vi "Combustion Stability Analysis.vi"() -> ()   [LabVIEW 2021]
uses:
  <vilib>/Utility/file.llb/Read Delimited Spreadsheet (string).vi
  <vilib>/Utility/file.llb/Read Delimited Spreadsheet (DBL).vi
panel:
  out "P-V Graph 3":cluster{" Total volume Vd":dbl[], dbl[]}(graph)
  out "Cycle Number":i32
  out "COV IMEP":dbl[](graph)
  out "COV Pmax":dbl[](graph)
  out "IMEP":dbl[](graph)
  out "P-V Graph 2":cluster{" Total volume Vd":dbl[], dbl[]}(graph)
  out "Data from file":dbl[][](array[numeric])
  out "CAmax per cycle":i32[](graph)
  out "CA(dp/dCA)max Graph":i32[](graph)
  out "(dp/dCA)max Graph  2":dbl[](graph)
  out "Pmax per cycle":dbl[](graph)
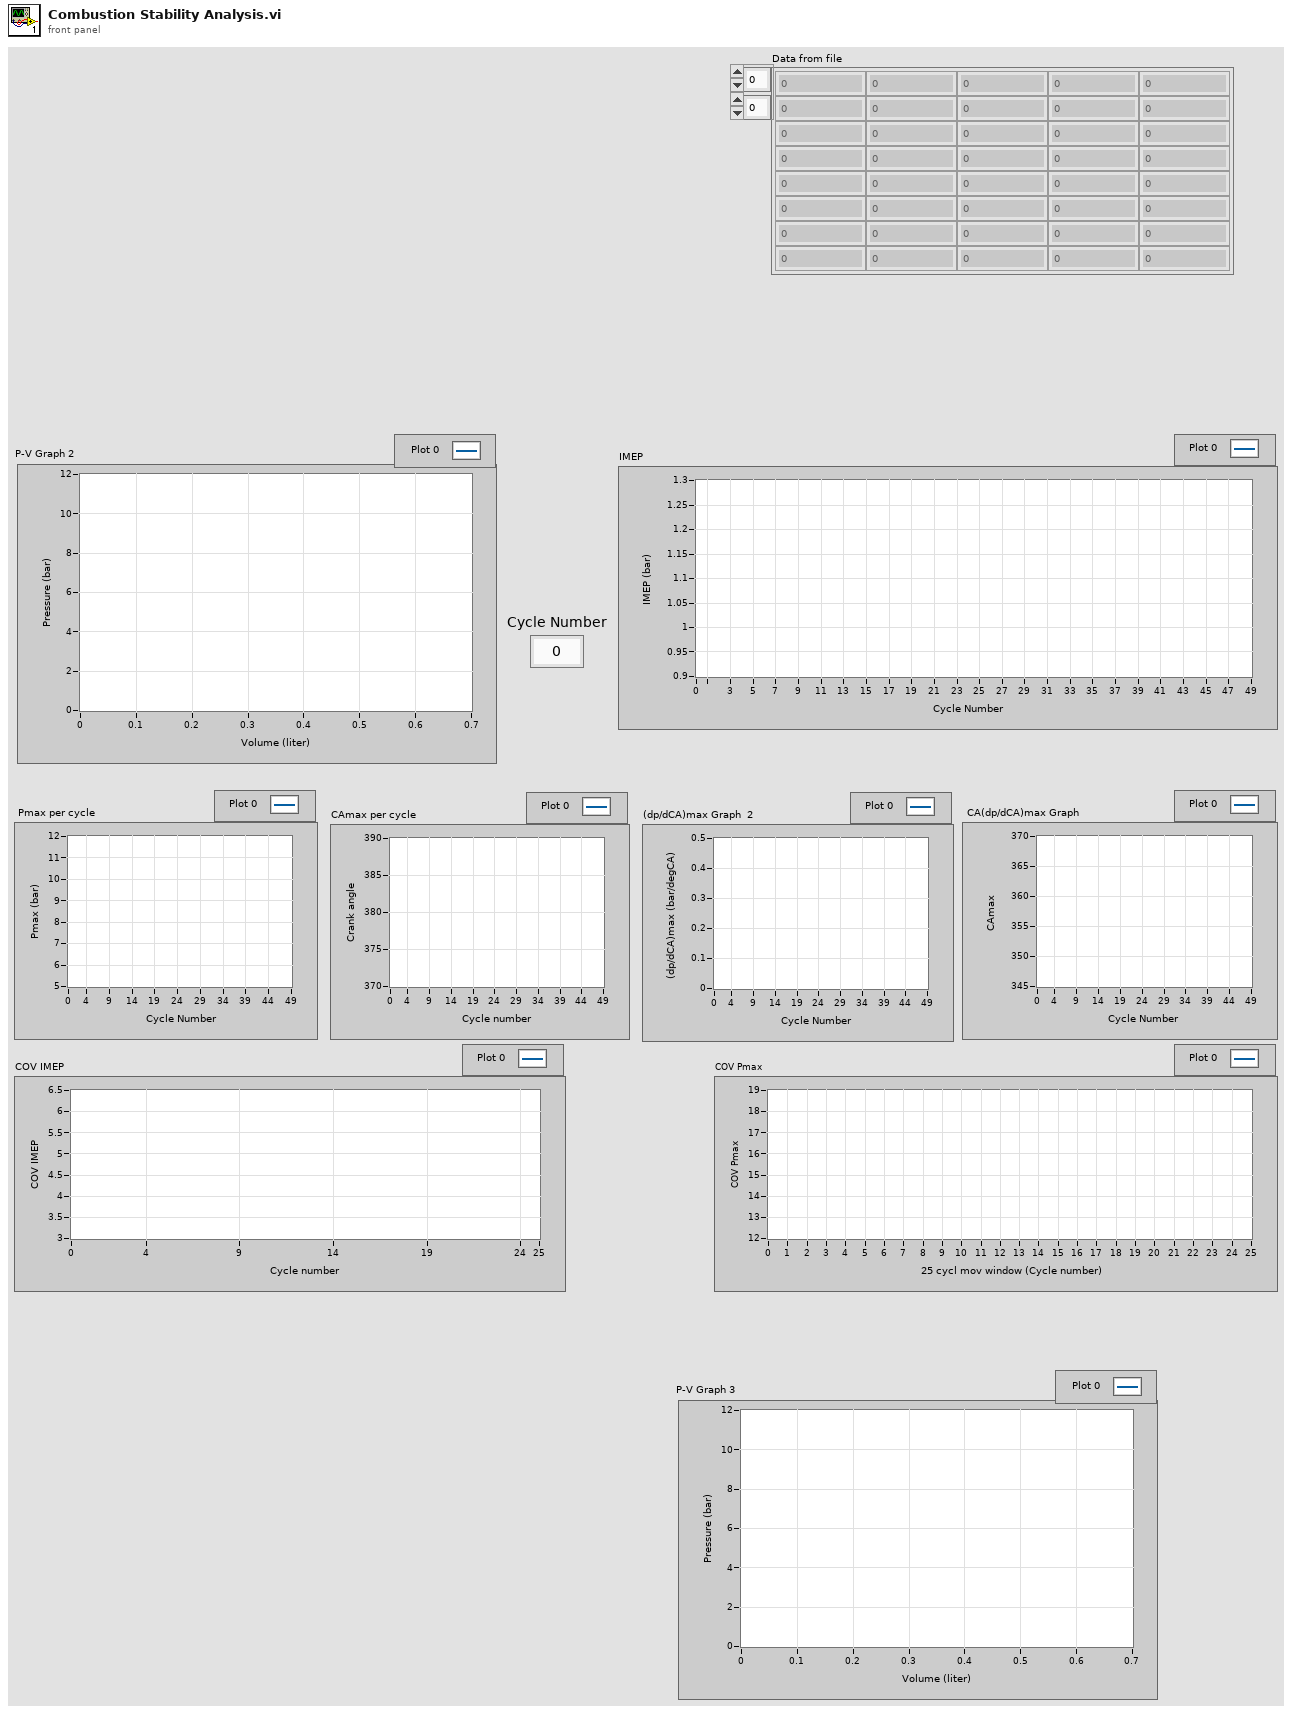
[diagram p1: front panel]
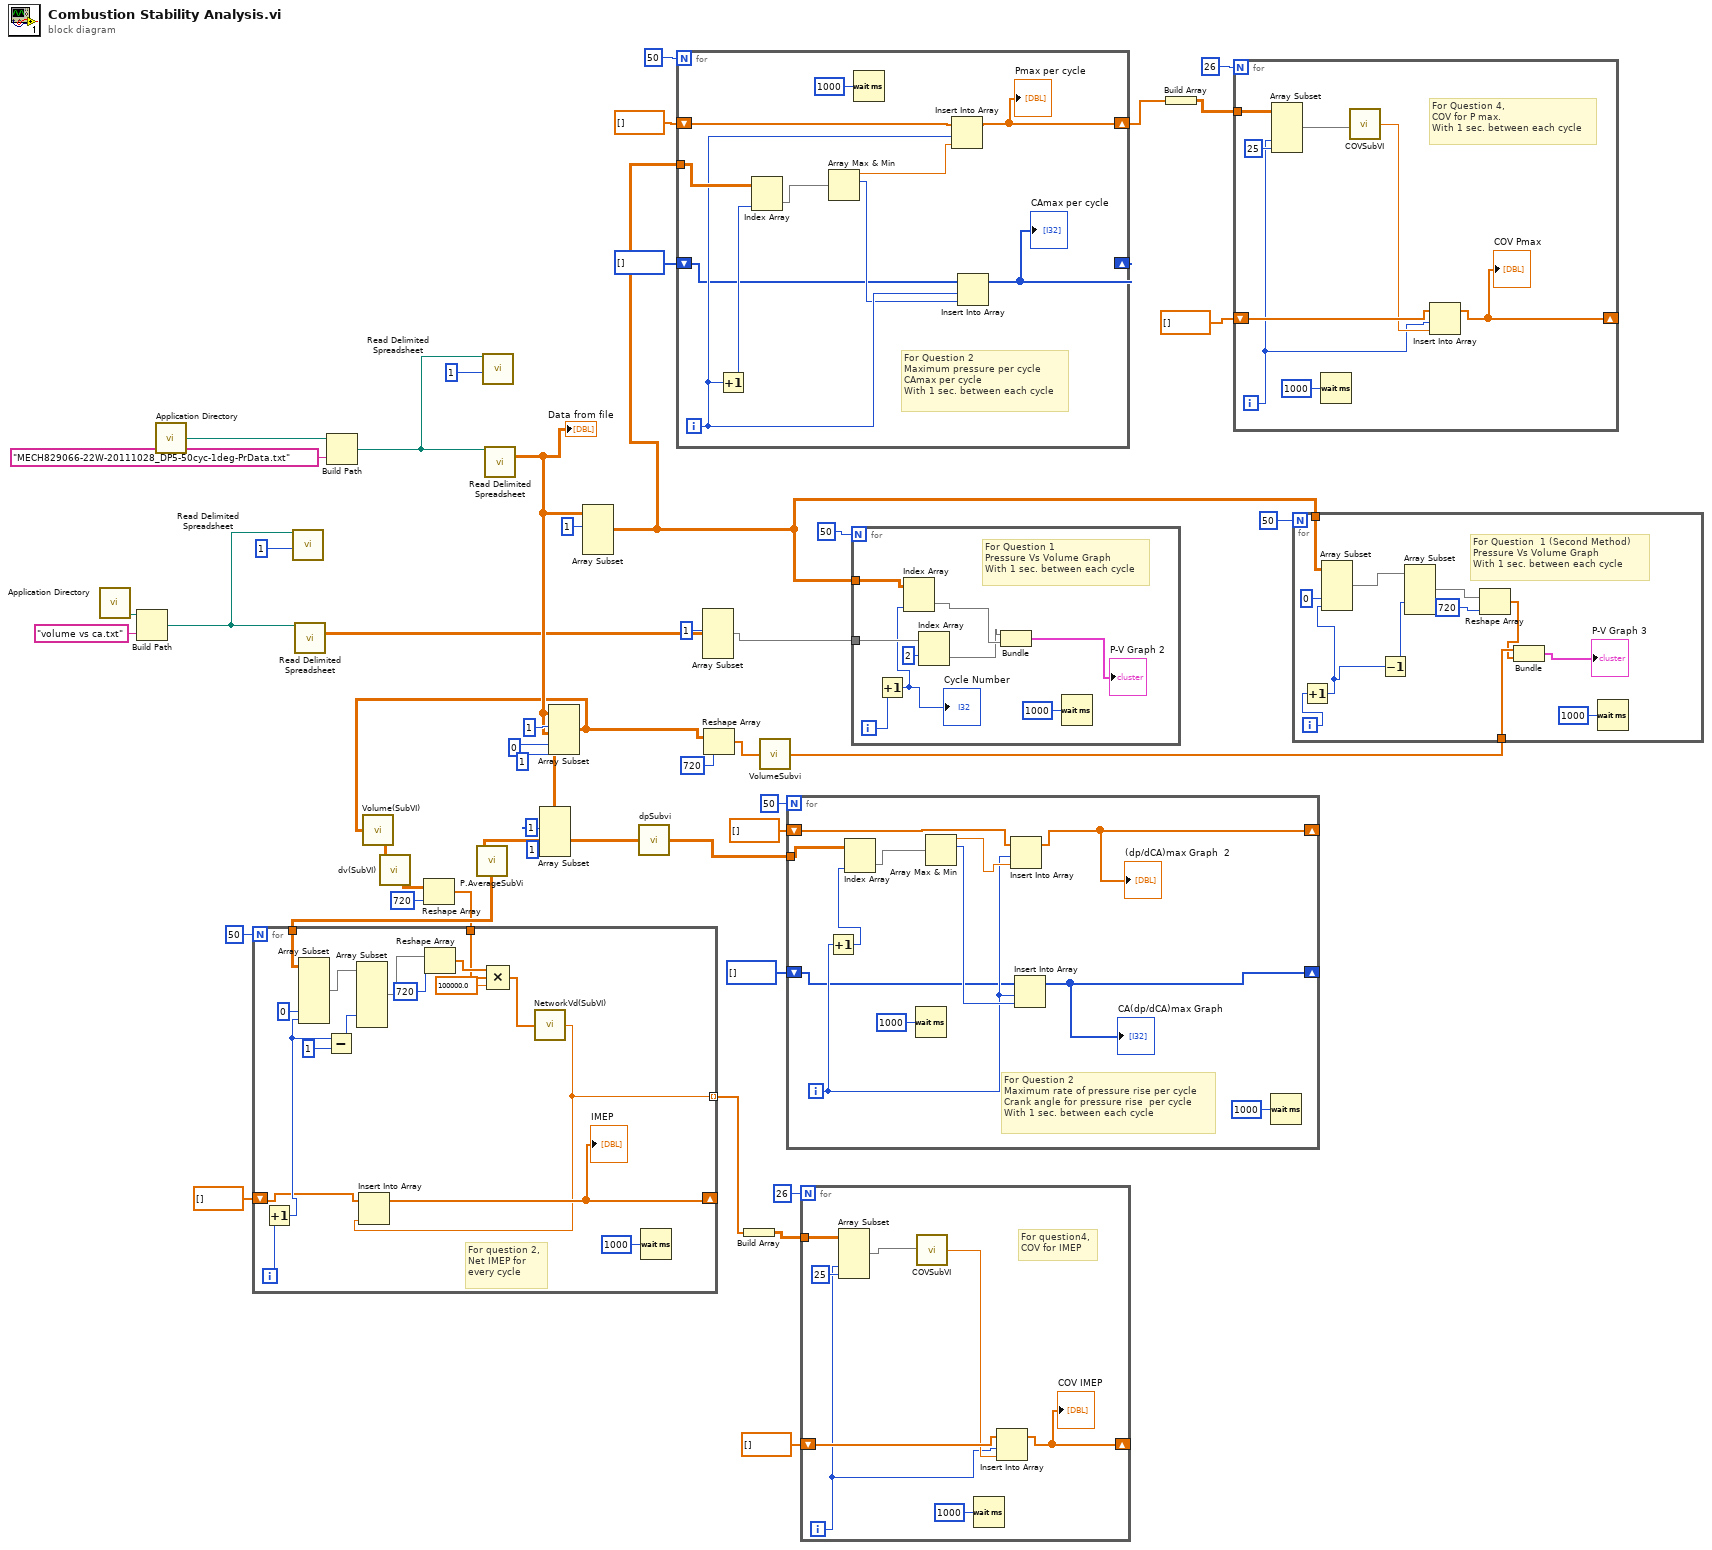
[diagram p0: block diagram]
diagram:
  n1 = call <vilib>:"Application Directory.vi"() -> ("Application Directory"=w25:path)
  n2 = Build Path(base path=w25, name or relative path="volume vs ca.txt") -> (appended path=w27:path)
  n3 = call <vilib>:"Application Directory.vi"() -> ("Application Directory"=w48:path)
  n4 = call-poly <vilib>:"Read Delimited Spreadsheet.vi"("file path (dialog if empty)"=w27, "number of rows (all:-1)"=1) -> ()  [unwired: 8 in, 6 out]
  n5 = call-poly <vilib>:"Read Delimited Spreadsheet.vi"("file path (dialog if empty)"=w27) -> ("all rows"=w24:dbl[][])  [unwired: 9 in, 5 out]
  n6 = Build Path(base path=w48, name or relative path="MECH829066-22W-20111028_DP5-50cyc-1deg-PrData.txt") -> (appended path=w46:path)
  n7 = call-poly <vilib>:"Read Delimited Spreadsheet.vi"("file path (dialog if empty)"=w46, "number of rows (all:-1)"=1) -> ()  [unwired: 8 in, 6 out]
  n8 = call-poly <vilib>:"Read Delimited Spreadsheet.vi"("file path (dialog if empty)"=w46) -> ("all rows"=w33:dbl[][])  [unwired: 9 in, 5 out]
  "Data from file" <- w33
  n9 = Array Subset "Array Subset"(array=w33, index (row)=1 ("index"), index (col)=1 ("index")) -> (w19:dbl[][])  [unwired: 2 in]
  n10 = call "P.AverageSubVi.vi"("Array"=w19) -> ("output array"=w30:dbl[][][])
  n11 = Array Subset "Array Subset"(array=w33, index (row)=1 ("index"), index (col)=0 ("index"), length (col)=1 ("length")) -> (w5:dbl[][])  [unwired: 1 in]
  n12 = call "Volume(SubVI).vi"("Array in"=w5) -> ("Array out"=w11:dbl[][])
  n13 = call "dv(SubVI).vi"("Array in"=w11) -> ("Array"=w10:dbl[][][])
  n14 = Reshape Array(w10, 720 ("dimension size")) -> (w8:dbl[])
  n15 = for {
    N: 50 -> [_]
    tunnel: w30 -> [w65]
    shift-right: [w52] -> _
    shift-left: dbl[] [] -> [w53]
    tunnel: [w51] -> w14 mode=indexing
    tunnel: w8 -> [w50]
    i -> [w63]
    # "For question 2,\nNet IMEP for\nevery cycle"
    n16 = Increment(x=w63) -> (x+1=w61:i32)
    n17 = Array Subset "Array Subset"(array=w65, index (dim 2)=0 ("index"), length (dim 2)=w61) -> (w62:dbl[][][])  [unwired: 4 in]
    n18 = Subtract(x=w61, y=1) -> (x-y=w60:i32)
    n19 = Array Subset(array=w62, index (dim 2)=w60) -> (w58:dbl[][][])  [unwired: 5 in]
    n20 = Reshape Array "Reshape Array"(w58, 720 ("dimension size")) -> (w55:dbl[])
    n21 = Compound Arithmetic op=MULTIPLY(w55, w50, 100000.0 ("value")) -> (w54:dbl[])
    n22 = call "NetworkVd(SubVI).vi"("Array"=w54) -> ("Numeric"=w51:dbl)
    n23 = Insert Into Array "Insert Into Array"(array=w53, new element=w51) -> (w52:dbl[])  [unwired: 1 in]
    "IMEP" <- w52
    n24 = Wait (ms)(milliseconds to wait=u32 1000) -> ()  [unwired: 1 out]
  }
  n25 = Array Subset "Array Subset"(array=w33, index (row)=1 ("index")) -> (w6:dbl[][])  [unwired: 3 in]
  n26 = call "dpSubvi.vi"("Array"=w19) -> ("output array"=w29:dbl[][])
  n27 = for {
    N: 50 -> [_]
    tunnel: w6 -> [w76]
    shift-right: [w72] -> w17
    shift-left: dbl[] [] -> [w73]
    shift-right: [w67] -> _
    shift-left: i32[] [] -> [w68]
    i -> [w70]
    # "For Question 2\nMaximum pressure per cycle\nCAmax per cycle\nWith 1 sec. between each cycle"
    n28 = Increment(x=w70) -> (x+1=w75:i32)
    n29 = Index Array "Index Array"(array=w76, index (col)=w75) -> (element=w74:dbl[])  [unwired: 1 in]
    n30 = Array Max & Min(array=w74) -> (max value=w71:dbl, max index (indices)=w69:i32)  [unwired: 2 out]
    n31 = Wait (ms)(milliseconds to wait=u32 1000) -> ()  [unwired: 1 out]
    n32 = Insert Into Array "Insert Into Array"(array=w73, index=w70, new element=w71) -> (w72:dbl[])
    "Pmax per cycle" <- w72
    n33 = Insert Into Array "Insert Into Array"(array=w68, index=w70, new element=w69) -> (w67:i32[])
    "CAmax per cycle" <- w67
  }
  n34 = Array Subset "Array Subset"(array=w24, index (row)=1 ("index")) -> (w22:dbl[][])  [unwired: 3 in]
  n35 = Reshape Array(w5, 720 ("dimension size")) -> (w3:dbl[])
  n36 = Build Array(w14) -> (w13:dbl[][])
  n37 = call "VolumeSubvi.vi"("Array"=w3) -> ("Total volume Vd"=w2:dbl[])
  n38 = for {
    N: 50 -> [_]
    shift-right: [w85] -> _
    shift-left: dbl[] [] -> [w86]
    shift-right: [w81] -> _
    shift-left: i32[] [] -> [w82]
    tunnel: w29 -> [w80]
    i -> [w83]
    # "For Question 2\nMaximum rate of pressure rise per cycle\nCrank angle for pressure rise  per cycle\nWith 1 sec. between each cycle"
    n39 = Increment(x=w83) -> (x+1=w79:i32)
    n40 = Index Array "Index Array"(array=w80, index (col)=w79) -> (element=w78:dbl[])  [unwired: 1 in]
    n41 = Wait (ms)(milliseconds to wait=u32 1000) -> ()  [unwired: 1 out]
    n42 = Array Max & Min(array=w78) -> (max value=w87:dbl, max index (indices)=w84:i32)  [unwired: 2 out]
    n43 = Insert Into Array "Insert Into Array"(array=w86, index=w83, new element=w87) -> (w85:dbl[])
    "(dp/dCA)max Graph  2" <- w85
    n44 = Insert Into Array "Insert Into Array"(array=w82, index=w83, new element=w84) -> (w81:i32[])
    "CA(dp/dCA)max Graph" <- w81
    n45 = Wait (ms)(milliseconds to wait=u32 1000) -> ()  [unwired: 1 out]
  }
  n46 = for {
    N: 26 -> [_]
    shift-right: [w93] -> _
    shift-left: dbl[] [] -> [w95]
    tunnel: w13 -> [w90]
    i -> [w91]
    # "For question4,\nCOV for IMEP"
    n47 = Array Subset "Array Subset"(array=w90, index (col)=w91, length (col)=25 ("length")) -> (w89:dbl[][])  [unwired: 2 in]
    n48 = call "COVSubVI.vi"("Array"=w89) -> ("Numeric"=w94:dbl)
    n49 = Wait (ms)(milliseconds to wait=u32 1000) -> ()  [unwired: 1 out]
    n50 = Insert Into Array(array=w95, index=w91, new element=w94) -> (w93:dbl[])
    "COV IMEP" <- w93
  }
  n51 = for {
    N: 50 -> [_]
    tunnel: w6 -> [w105]
    tunnel: w22 -> [w100]
    i -> [w104]
    # "For Question 1\nPressure Vs Volume Graph\nWith 1 sec. between each cycle"
    n52 = Increment(x=w104) -> (x+1=w97:i32)
    "Cycle Number" <- w97
    n53 = Index Array "Index Array"(array=w105, index (col)=w97) -> (element=w102:dbl[])  [unwired: 1 in]
    n54 = Index Array(array=w100, index (col)=2) -> (element=w101:dbl[])  [unwired: 1 in]
    n55 = Bundle(w101, w102) -> (→"P-V Graph 2":cluster{dbl[], dbl[]})  [unwired: 1 in]
    n56 = Wait (ms)(milliseconds to wait=u32 1000) -> ()  [unwired: 1 out]
  }
  n57 = Build Array(w17) -> (w16:dbl[][])
  n58 = for {
    N: 26 -> [_]
    tunnel: w16 -> [w113]
    shift-right: [w108] -> _
    shift-left: dbl[] [] -> [w110]
    i -> [w106]
    # "For Question 4,\nCOV for P max.\nWith 1 sec. between each cycle"
    n59 = Array Subset(array=w113, index (col)=w106, length (col)=25 ("length")) -> (w111:dbl[][])  [unwired: 2 in]
    n60 = Wait (ms)(milliseconds to wait=u32 1000) -> ()  [unwired: 1 out]
    n61 = call "COVSubVI.vi"("Array"=w111) -> ("Numeric"=w109:dbl)
    n62 = Insert Into Array(array=w110, index=w106, new element=w109) -> (w108:dbl[])
    "COV Pmax" <- w108
  }
  n63 = for {
    N: 50 -> [_]
    tunnel: w6 -> [w125]
    tunnel: w2 -> [w119]
    i -> [w123]
    # "For Question  1 (Second Method)\nPressure Vs Volume Graph\nWith 1 sec. between each cycle"
    n64 = Increment(x=w123) -> (x+1=w121:i32)
    n65 = Array Subset "Array Subset"(array=w125, index (col)=0 ("index"), length (col)=w121) -> (w122:dbl[][])  [unwired: 2 in]
    n66 = Decrement(x=w121) -> (x-1=w120:i32)
    n67 = Array Subset "Array Subset"(array=w122, index (col)=w120) -> (w117:dbl[][])  [unwired: 3 in]
    n68 = Reshape Array(w117, 720 ("dimension size")) -> (w116:dbl[])
    n69 = Bundle("Total volume Vd"=w119, w116) -> (→"P-V Graph 3":cluster{" Total volume Vd":dbl[], dbl[]})  [unwired: 1 in]
    n70 = Wait (ms)(milliseconds to wait=u32 1000) -> ()  [unwired: 1 out]
  }
